vi "Move Tuner per Gamma.vi"(8 "error in (no error)":errorcluster, 9 "Timeout (60 s)":u8=60, 10 "Gamma":cdb, 11 "iTuner reference in":refnum<k7>) -> (0 "error out":errorcluster, 2 "Current Gammas":cdb[](array[numeric]), 3 "iTuner reference out":refnum<k7>)   [LabVIEW 2016, in "FocusTuner.lvlib"]
doc: "Sets the specified reflection coefficient in the device reference plane at fundamental frequency with timeout."
uses:
  FocusTuner.lvlib
  <instrlib>/Focus iTuner Series/Public/Action-Status/Move Tuner per Reflection Coefficient (Main Section).vi
  <instrlib>/Focus iTuner Series/Public/Data/Query Reflection Coefficient (Current Position - All Frequencies).vi
  <instrlib>/Focus iTuner Series/Focus iTuner Series.lvlib
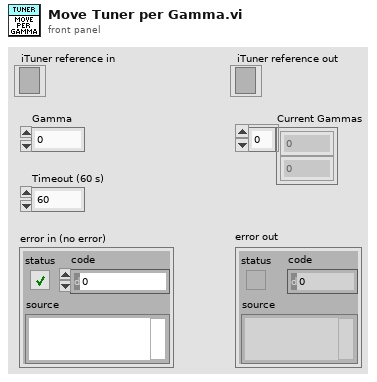
[diagram p1: front panel]
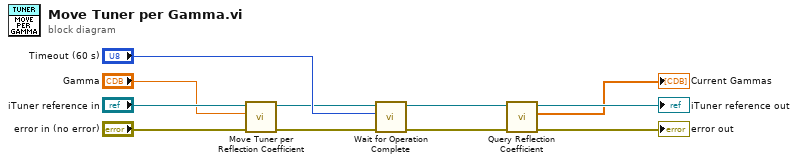
[diagram p0: block diagram]
diagram:
  n1 = call-poly <instrlib>:"Move Tuner per Reflection Coefficient.vi"("error in (no error)"="error in (no error)", "Reflection Coefficient"="Gamma", "iTuner reference in"="iTuner reference in") -> ("error out"=w3:errorcluster, "iTuner reference out"=w4:refnum<k7>)  [unwired: 7 in]
  n2 = call <instrlib>:"Wait for Operation Complete.vi"("error in (no error)"=w3, "Timeout (60 s)"="Timeout (60 s)", "iTuner reference in"=w4) -> ("error out"=w1:errorcluster, "iTuner reference out"=w2:refnum<k7>)  [unwired: 7 in]
  n3 = call-poly <instrlib>:"Query Reflection Coefficient.vi"("error in (no error)"=w1, "iTuner reference in"=w2) -> ("error out"=→"error out":errorcluster, "Reflection Coefficients"=→"Current Gammas":cdb[], "iTuner reference out"=→"iTuner reference out":refnum<k7>)  [unwired: 7 in]
